vi "RT_Call Check Idle.vi"(6 "Timeout?":i32=1000, 8 "error in":errorcluster, 11 "FPGA VI Reference In":T1) -> (0 "error out":errorcluster, 3 "FPGA VI Reference Out":T1)   [LabVIEW 2018]
uses:
  Data Def/RT_FPGA VI Reference.ctl
  <vilib>/Utility/error.llb/Error Cluster From Error Code.vi
  <vilib>/rvi/errors/niLvFpgaAdjustHostInterfaceError.vi
  <vilib>/rvi/interface/nirviReadWriteControl/nirviReadWriteControl.xnode
  NiFpgaLv.dll
  <vilib>/rvi/interface/Simulation/niFpgaSimulationCallBeginRW.vi
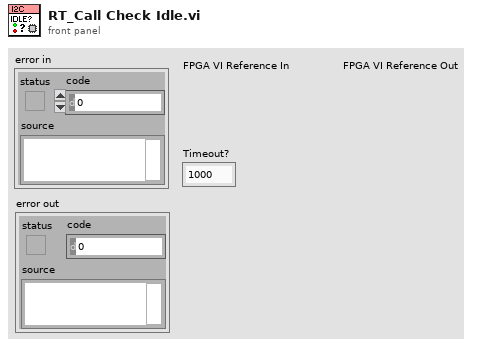
[diagram p1: front panel]
types:
  T1 = typedef "RT_FPGA VI Reference.ctl" = refnum<k20>
  T2 = enum16{"Idle", "Set Idle", "Config", "Read", "Write", "Arm", "Auto Run", "Auto Config", "Auto Write", "Auto Arm", "Auto Read", "Auto Check"}
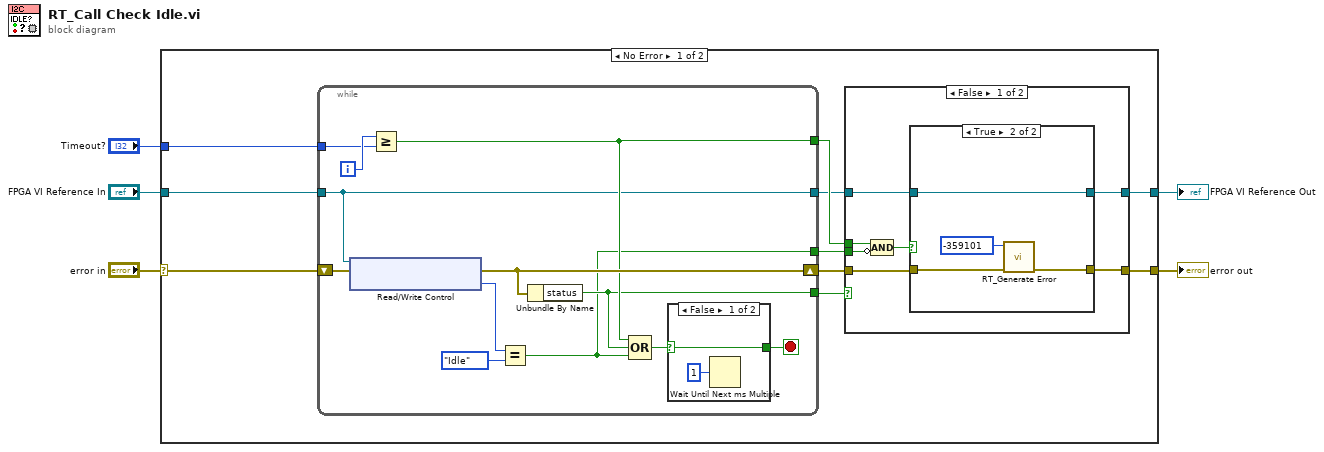
[diagram p0: block diagram]
diagram:
  n1 = case shown="No Error" "error in" {
    selector: "error in" -> [w14 w47]
    tunnel: [w15 w47] -> w5
    tunnel: "Timeout?" -> [w6 _]
    tunnel: "FPGA VI Reference In" -> [w13 w46]
    tunnel: [w7 w46] -> w1
    frame No Error {
      n2 = while {
        shift-right: [w41] -> w12
        shift-left: w14 -> [w42]
        tunnel: [w35] -> w8
        tunnel: w13 -> [w35]
        tunnel: w6 -> [w32]
        tunnel: [w40] -> w9
        tunnel: [w36] -> w10
        tunnel: [w37] -> w11
        i -> [w33]
        stop <- w38 stop-if-true
        n3 = xnode "Read/Write Control"("FPGA VI Reference In"=w35, "error in"=w42) -> ("error out"=w41:errorcluster, "I2C Loop State View"=w34:T2)  [unwired: 1 out]
        n4 = Greater Or Equal?(x=w33, y=w32) -> (x >= y?=w40:bool)
        n5 = Equal?(x=w34, y=T2."Idle") -> (x = y?=w36:bool)
        n6 = Unbundle By Name(w41) -> ("status"=w37:bool)
        n7 = Compound Arithmetic op=OR(w40, w37, w36) -> (w39:bool)
        n8 = case shown="False" w39 {
          selector: w39 -> [w44 w45]
          tunnel: [w44 w45] -> w38
          frame False {
            n9 = Wait Until Next ms Multiple(millisecond multiple=u32 1) -> ()  [unwired: 1 out]
          }
          frame True {
          }
        }
      }
      n10 = case shown="False" w11 {
        tunnel: w12 -> [w22 w30]
        tunnel: [w21 w30] -> w15
        tunnel: w10 -> [w20 _]
        tunnel: w9 -> [w18 _]
        tunnel: w8 -> [w17 w29]
        tunnel: [w16 w29] -> w7
        frame False {
          n11 = Compound Arithmetic op=AND(w18, invert w20) -> (w19:bool)
          n12 = case shown="True" w19 {
            tunnel: w22 -> [w24 w28]
            tunnel: [w24 w27] -> w21
            tunnel: w17 -> [w23 w25]
            tunnel: [w23 w25] -> w16
            frame False {
            }
            frame True {
              n13 = call "RT_Generate Error.vi"("error in (no error)"=w28, "Code"=-359101) -> ("error out"=w27:errorcluster)  [unwired: 9 in]
            }
          }
        }
        frame True {
        }
      }
    }
    frame Error {
    }
  }
  "error out" <- w5
  "FPGA VI Reference Out" <- w1
